vi "Auton Rotate.vi"(0 "Rotation":dbl=3.0 format="%#_13g", 1 "PID gains":T1 {"derivative time (Td, min)" format="%.3f"; "integral time (Ti, min)" format="%.3f"; "proportional gain (Kc)" format="%.3f"}, 2 "PID Complete Delay":u32, 3 "Refnum in":refnum<k33>) -> (7 "Degrees Rotated":dbl, 10 "rt fifo out":refnum<k33>)   [LabVIEW 2014]
uses:
  TeleopCmd.ctl
  CmdFlag.ctl
  AutonCals.vi
  <vilib>/addons/control/pid/pid.llb/PID (DBL).vi
  <vilib>/addons/control/pid/NI_PID_pid.lvlib
panel:
  out "dt out (s)":dbl format="%.3f"
  out "PID output":dbl format="%.2f"
  out "Moving slow":bool
  out "Close to goal":bool
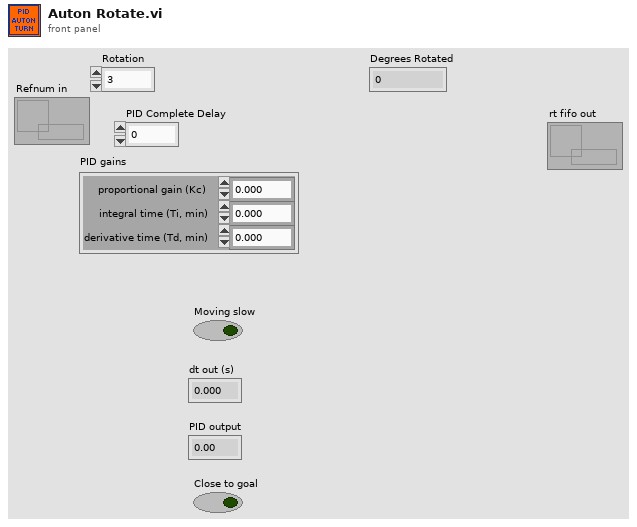
[diagram p1: front panel]
types:
  T1 = cluster{"proportional gain (Kc)":dbl, "integral time (Ti, min)":dbl, "derivative time (Td, min)":dbl}
  T2 = typedef "TeleopCmd.ctl" = cluster{"CmdFlag":T3, "throttle":dbl, "turn":dbl, "Override":bool, "Strafe":dbl, "MotorPwrMax":u8, "Time":u32, "ultrasonic override":bool}
  T3 = typedef "CmdFlag.ctl" = enum16{"noop", "logflag", "suspend", "resume"}
  T4 = typedef "navX-MXP IMU.lvlib/navX YPRH Data.ctl" = cluster{"Yaw":dbl, "Pitch":dbl, "Roll":dbl, "Heading":dbl}
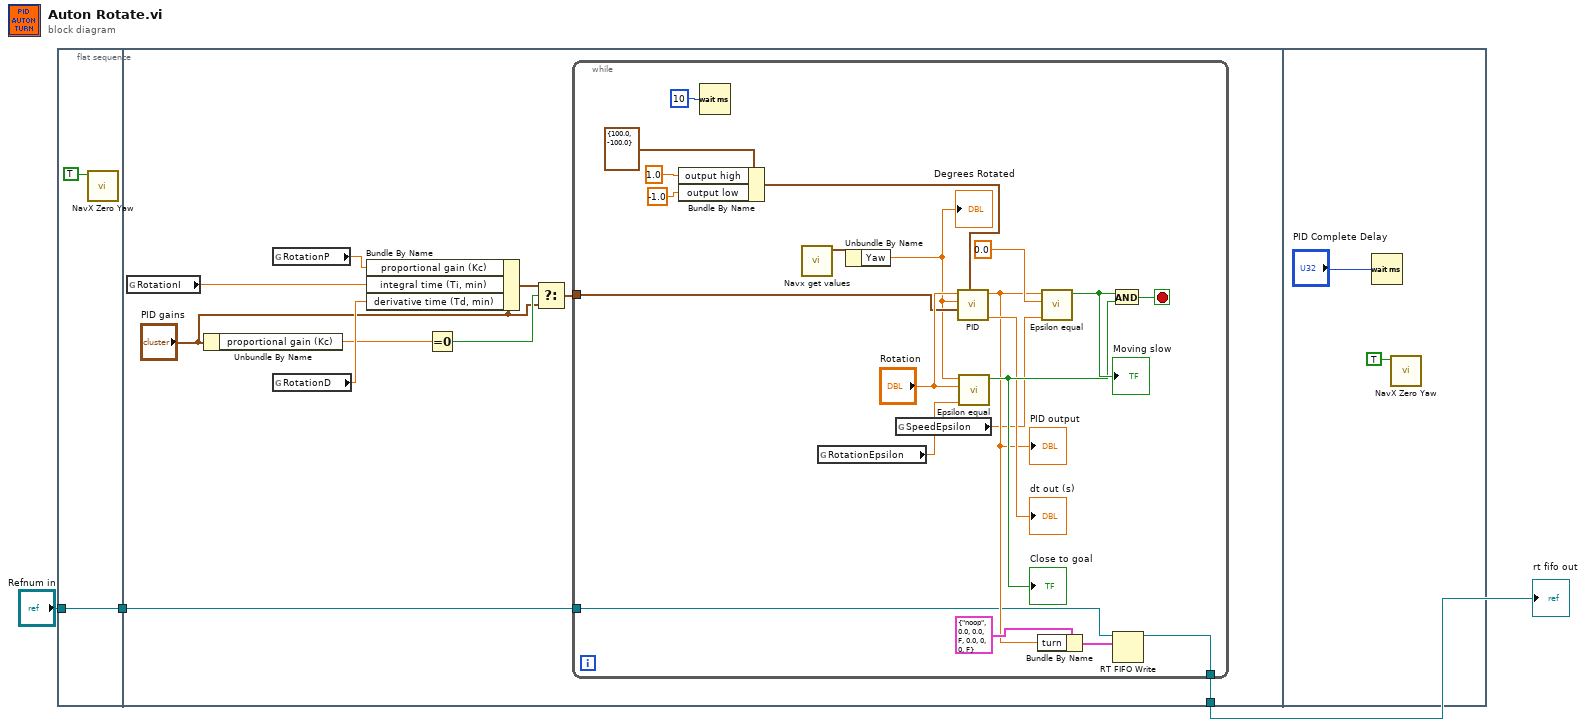
[diagram p0: block diagram]
diagram:
  n1 = flat-sequence {
    tunnel: "Refnum in" -> [w5]
    tunnel: [w5] -> w1
    tunnel: [w6] -> w2
    tunnel: w1 -> [w15]
    frame #0 {
      n2 = call "NavX Zero Yaw.vi"("Reset NavX Yaw"=TRUE) -> ()  [unwired: 11 in]
    }
    frame #1 {
      n3 = global read "AutonCals.vi" "RotationI"() -> (w14:dbl)
      n4 = Unbundle By Name("PID gains") -> ("proportional gain (Kc)"=w10:dbl)
      n5 = global read "AutonCals.vi" "RotationP"() -> (w12:dbl)
      n6 = global read "AutonCals.vi" "RotationD"() -> (w13:dbl)
      n7 = Bundle By Name(cluster="PID gains", "proportional gain (Kc)"=w12, "integral time (Ti, min)"=w14, "derivative time (Td, min)"=w13) -> (w9:T1)
      n8 = Equal To 0?(x=w10) -> (x = 0?=w11:bool)
      n9 = Select(t=w9, s=w11, f="PID gains") -> (s? t:f=w7:T1)
      n10 = while {
        tunnel: w15 -> [w24]
        tunnel: w7 -> [w19]
        tunnel: [w18] -> w6
        stop <- w31 stop-if-true
        n11 = Bundle By Name(cluster=cluster{"output high":dbl, "output low":dbl} {"output high"=100.0, "output low"=-100.0} ("output range"), "output high"=1.0, "output low"=-1.0) -> (w35:cluster{"output high":dbl, "output low":dbl})
        n12 = Wait (ms)(milliseconds to wait=u32 10) -> ()  [unwired: 1 out]
        n13 = call "Navx get values.vi"() -> ("YPRH"=w17:T4)  [unwired: 11 in]
        n14 = global read "AutonCals.vi" "RotationEpsilon"() -> (w22:dbl)
        n15 = Unbundle By Name(w17) -> ("Yaw"=w16:dbl)
        "Degrees Rotated" <- w16
        n16 = global read "AutonCals.vi" "SpeedEpsilon"() -> (w21:dbl)
        n17 = call-poly <vilib>:"PID.vi"("output range"=w35, "PID gains"=w19, "process variable"=w16, "setpoint"="Rotation") -> ("dt out (s)"=→"dt out (s)":dbl, "output"=w26:dbl)  [unwired: 6 in]
        "PID output" <- w26
        n18 = call "Epsilon equal.vi"("Epsilon"=w22, "Value2"="Rotation", "Value1"=w16) -> ("Boolean"=w29:bool)  [unwired: 8 in]
        "Close to goal" <- w29
        n19 = Bundle By Name(cluster=T2 {"CmdFlag"=enum."noop", "throttle"=0.0, "turn"=0.0, "Override"=FALSE, "Strafe"=0.0, "MotorPwrMax"=0, "Time"=0, "ultrasonic override"=FALSE} ("Cluster"), "turn"=w26) -> (w25:T2)
        n20 = call "Epsilon equal.vi"("Epsilon"=w21, "Value2"=0.0, "Value1"=w26) -> ("Boolean"=w30:bool)  [unwired: 8 in]
        "Moving slow" <- w30
        n21 = And(x=w30, y=w29) -> (x .and. y?=w31:bool)
        n22 = RT FIFO Write(0:w24, 1:w25) -> (8:w18:refnum<k33>)  [unwired: 3 in, 3 out]
      }
    }
    frame #2 {
      n23 = Wait (ms)(milliseconds to wait="PID Complete Delay") -> ()  [unwired: 1 out]
      n24 = call "NavX Zero Yaw.vi"("Reset NavX Yaw"=TRUE) -> ()  [unwired: 11 in]
    }
  }
  "rt fifo out" <- w2
